vi "CCSaveDICOMValuesToFile.vi"(8 "error in (no error)":errorcluster, 10 "DICOM Values":string[](array[string]), 11 "File Dest":string) -> (0 "error out":errorcluster, 2 "Save":bool)   [LabVIEW 2013, in "ClearCanvasLibrary.lvlib"]
uses:
  Controls/Enum Variables.ctl
  C:/Users/Simon/SkyDrive/LabView/2013/DM2020/DICOM/ClearCanvasNewBuild/ClearCanvas.Dicom.dll
  ClearCanvasNewBuild/ClearCanvas.Dicom.dll
  <userlib>/_OpenG.lib/file/file.llb/File Exists - Scalar__ogtk.vi
  <userlib>/_MGI/Error Handling/MGI Suppress Error Code/MGI Suppress Error Code (Scalar).vi
  ClearCanvasLibrary.lvlib
  main.lvlib
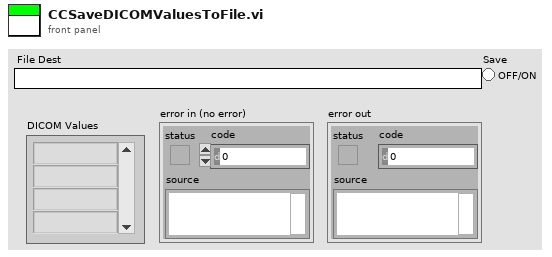
[diagram p1: front panel]
types:
  T1 = typedef "main.lvlib/Enum Variables.ctl" = enum16{"SetAcqFilter", "GetAcqFilter", "Set Filter", "Get Filter", "Set Height", "Get Height", "Set Blue Pressure", "Get Blue Pressure", "Set Red Pressure", "Get Red Pressure", "Init", "Reset Pressure", "Set Red Cursors", "Get Red Cursors", "Set Blue Cursors", "Get Blue Cursors", "Set Language", "Get Language", "Set Active Graphs", "Get ActiveGraphs", "Set Method", "Get Method", "Set Encryption", "Get Encryption", "Set ExcelVersion", "Get ExcelVersion", "Set itemTags", "Get itemTags", "Set Attributes", "Get Attributes", "Set DICOM Avail", "Get DICOM Avail", "Set DICOM Encode", "Get DICOM Encode", "Set JournalExport", "Get JournalExport", "Set Sequence", "Get Sequence", "Set DAQ Connected", "Get DAQ Connected", "Set Current Graph", "Get Current Graph", "Set General Settings", "Get Hyphenation", "Set Arm Calc Method", "Get Arm Calc Method", "Set Dicom Tags", "Get Dicom Tags"}
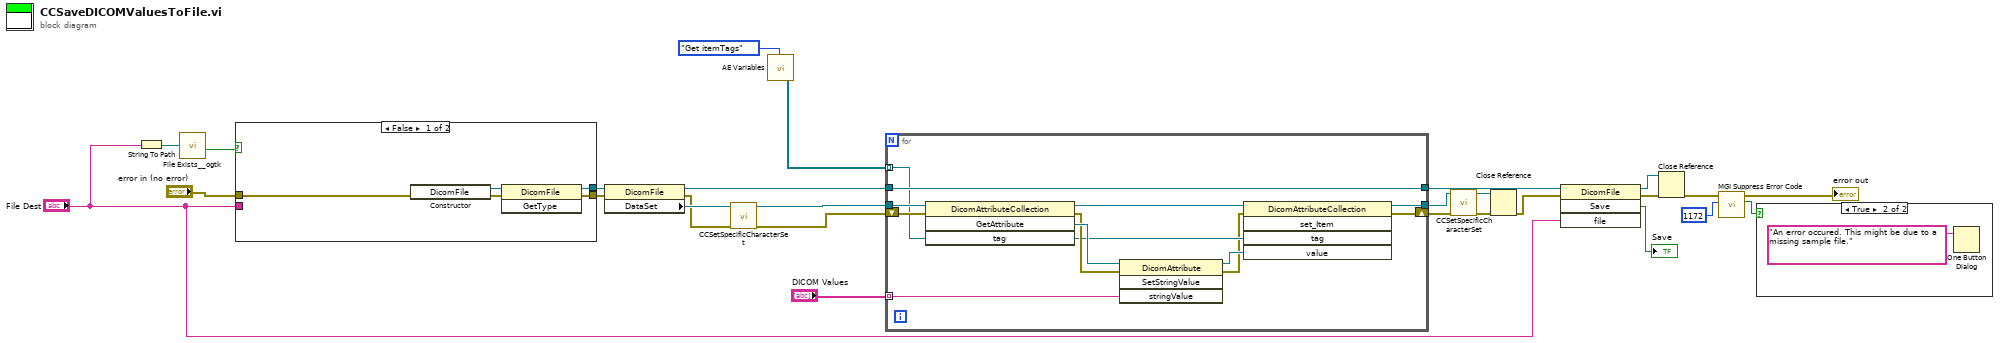
[diagram p0: block diagram]
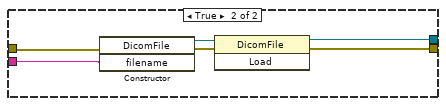
[diagram p3: hidden frame]
diagram:
  n1 = String To Path(string="File Dest") -> (path=w19:path)
  n2 = call-poly <userlib>:"File Exists__ogtk.vi"("file path"=w19) -> ("exists"=w6:bool)  [unwired: 6 in, 1 out]
  n3 = case shown="False" w6 {
    tunnel: "error in (no error)" -> [w32 w34]
    tunnel: [w28 w38] -> w21
    tunnel: [w29 w37] -> w20
    tunnel: "File Dest" -> [_ w33]
    frame False {
      n4 = constructor class="DicomFile"(error in=w32) -> (reference out=w31:refnum<k24>, error out=w30:errorcluster)  [unwired: 2 in, 1 out]
      n5 = invoke class="DicomFile" method="GetType"(reference=w31, error in=w30) -> (reference out=w28:refnum<k24>, error out=w29:errorcluster)  [unwired: 1 in, 1 out]
    }
    frame True {
      n6 = constructor class="DicomFile"(error in=w34, "filename"=w33) -> (reference out=w36:refnum<k24>, error out=w35:errorcluster)  [unwired: 2 in, 2 out]
      n7 = invoke class="DicomFile" method="Load"(reference=w36, error in=w35) -> (reference out=w38:refnum<k24>, error out=w37:errorcluster)  [unwired: 1 in, 1 out]
    }
  }
  n8 = property class="DicomFile"(reference=w21, error in=w20) -> (reference out=w11:refnum<k24>, error out=w7:errorcluster, "DataSet"=w10:refnum<k24>)
  n9 = call "CCSetSpecificCharacterSet.vi"("error in (no error)"=w7, ".NET Refnum in"=w10) -> ("error out"=w9:errorcluster, ".NET Refnum out"=w8:refnum<k24>)  [unwired: 8 in]
  n10 = call "AE Variables.vi"("Action"=Enum_Variables."Get itemTags") -> ("itemTags .net"=w14:refnum<k24>[])  [unwired: 10 in, 8 out]
  n11 = for {
    tunnel: w8 -> [w47]
    tunnel: w11 -> [w48]
    tunnel: [w48] -> w26
    shift-right: [w50] -> w4
    shift-left: w9 -> [w46]
    tunnel: [w49] -> w1
    tunnel: w14 -> [w41] mode=indexing
    tunnel: "DICOM Values" -> [w40] mode=indexing
    n12 = invoke class="DicomAttributeCollection" method="GetAttribute"(reference=w47, error in=w46, "tag"=w41) -> (reference out=w45:refnum<k24>, error out=w43:errorcluster, "GetAttribute"=w44:refnum<k24>)  [unwired: 1 in, 1 out]
    n13 = invoke class="DicomAttribute" method="SetStringValue"(reference=w44, error in=w43, "stringValue"=w40) -> (reference out=w42:refnum<k24>, error out=w39:errorcluster)  [unwired: 1 in, 2 out]
    n14 = invoke class="DicomAttributeCollection" method="set_Item"(reference=w45, error in=w39, "tag"=w41, "value"=w42) -> (reference out=w49:refnum<k24>, error out=w50:errorcluster)  [unwired: 1 in, 3 out]
  }
  n15 = call "CCSetSpecificCharacterSet.vi"("error in (no error)"=w4, ".NET Refnum in"=w1) -> ("error out"=w3:errorcluster, ".NET Refnum out"=w2:refnum<k24>)  [unwired: 8 in]
  n16 = Close Reference(reference=w2, error in (no error)=w3) -> (error out=w23:errorcluster)
  n17 = invoke class="DicomFile" method="Save"(reference=w26, error in=w23, "file"="File Dest") -> (reference out=w24:refnum<k24>, error out=w25:errorcluster, "Save"=→"Save":bool)  [unwired: 1 in, 1 out]
  n18 = Close Reference(reference=w24, error in (no error)=w25) -> (error out=w18:errorcluster)
  n19 = call-poly <userlib>:"MGI Suppress Error Code.vi"("Error Code"=1172, "Error In"=w18) -> ("Error Supressed?"=w15:bool, "Error Out"=→"error out":errorcluster)  [unwired: 4 in]
  n20 = case shown="True" w15 {
    frame False {
    }
    frame True {
      n21 = One Button Dialog(message="An error occured. This might be due to a missing sample file.") -> ()  [unwired: 1 in, 1 out]
    }
  }
